vi "Robot Global Data.vi"() -> ()   [LabVIEW 2014]
doc: "This global VI can contain as many global variables as you need. Place a control on the panel, give it a good name. To read or write to it from a VI, drag the icon to the diagram of that VI. You can also drag from the project. Click on the node to change which global you access. You shouldn't have multiple locations writing to a global or it will cause a race-condition."
uses:
  <vilib>/Rock Robotics/WPI/Camera/WPI_CameraImageSize.ctl
  <vilib>/Rock Robotics/WPI/DriverStation/WPI_DriverStationRobotMode2.ctl
panel:
  in  "Autonomous":T1
  out "Secondary Controller":T2
  out "Tote in front?":bool
  out "Sensors":T3
  in  "Lift Position":dbl
  in  "Clamp Position":dbl
  in  "Robot Mode":T4
  in  "image size":T5=enum."320x240"
  in  "Enable Vision":bool
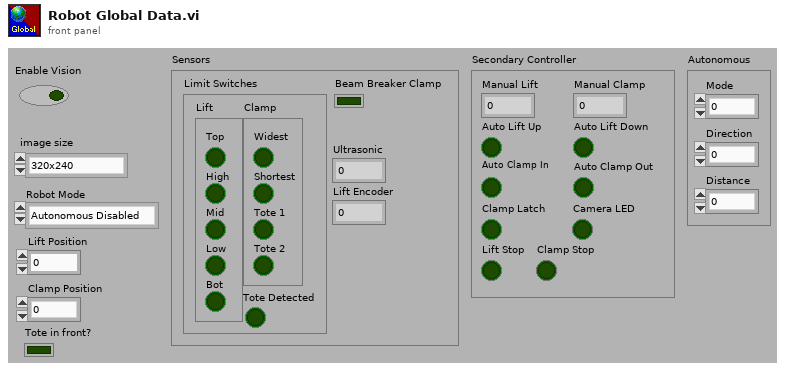
[diagram p1: front panel]
types:
  T1 = cluster{"Mode":dbl, "Direction":dbl, "Distance":dbl}
  T2 = cluster{"Manual Lift":dbl, "Manual Clamp":dbl, "Auto Lift Up":bool, "Auto Lift Down":bool, "Auto Clamp In":bool, "Auto Clamp Out":bool, "Clamp Latch":bool, "Camera LED":bool, "Lift Stop":bool, "Clamp Stop":bool}
  T3 = cluster{"Limit Switches":cluster{"Lift":cluster{"Top":bool, "High":bool, "Mid":bool, "Low":bool, "Bot":bool}, "Clamp":cluster{"Widest":bool, "Shortest":bool, "Tote 1":bool, "Tote 2":bool}, "Tote Detected":bool}, "Ultrasonic":dbl, "Beam Breaker Clamp":bool, "Lift Encoder":dbl}
  T4 = typedef "WPI_DriverStationRobotMode2.ctl" = enum16{"Autonomous Disabled", "Autonomous Enabled", "Teleop Disabled", "Teleop Enabled", "Disconnected", "Finish", "Test Disabled", "Test Enabled", "Emergency Stopped"}
  T5 = typedef "WPI_CameraImageSize.ctl" = enum16{"640x480", "320x240", "160x120", "Custom"}
diagram:
